vi "AES-InvCipher-text.vi"(5 "Initializer Vector":u8[](array[numeric]), 7 "Operation Mode":T1, 8 "error in (no error)":errorcluster, 10 "Cipher Key":u8[](array[numeric]), 11 "ciphertext":u8[](array[numeric])) -> (0 "error out":errorcluster, 3 "plaintext":u8[](array[numeric]))   [LabVIEW 2011, in "i3-external-encryption.lvlib"]
doc: "Decripts the <b>ciphertext</b> by using the cipher and the given <b>Operation Mode</b> using AES algorithm.\nThe cipher key and initialization vector should be a hex-string (ASCII values 0-f).\nCAUTION:\nThis VI is not secure, it does not protect the memory of the encryption, key and unencrypted data.\n\n(c) Ton Plomp, 2011\nTHIS SOFTWARE IS PROVIDED AS IS, AND ANY WARRANTY IS REJECTED"
uses:
  i3-external-encryption.lvlib
  AES-Modes.ctl
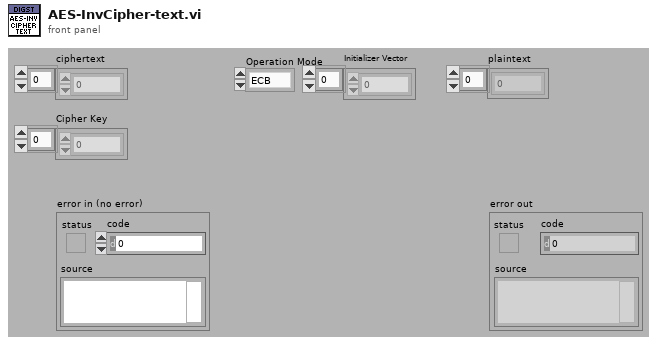
[diagram p1: front panel]
types:
  T1 = typedef "i3-external-encryption.lvlib/AES-Modes.ctl" = enum16{"ECB", "CBC", "CFB128", "OFB"}
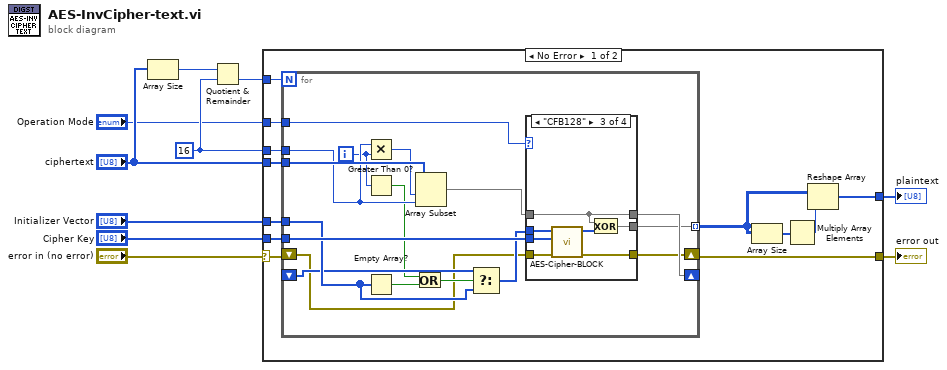
[diagram p0: block diagram]
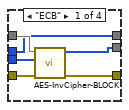
[diagram p2: hidden frame]
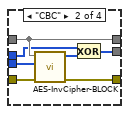
[diagram p3: hidden frame]
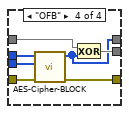
[diagram p4: hidden frame]
diagram:
  w6 = 16 ("y")
  n1 = Array Size(array="ciphertext") -> (size(s)=w8:i32)
  n2 = Quotient & Remainder(x=w8, y=w6) -> (floor(x/y)=w5:i32)  [unwired: 1 out]
  n3 = case shown="No Error" "error in (no error)" {
    selector: "error in (no error)" -> [w18 w67]
    tunnel: "ciphertext" -> [w22 _]
    tunnel: [w17 w67] -> w9
    tunnel: "Cipher Key" -> [w21 _]
    tunnel: w5 -> [w20 _]
    tunnel: w6 -> [w19 _]
    tunnel: [w11 _] -> w7
    tunnel: "Initializer Vector" -> [w15 _]
    tunnel: "Operation Mode" -> [w16 _]
    frame No Error {
      n4 = for {
        N: w20 -> [_]
        tunnel: w22 -> [w38]
        tunnel: w21 -> [w39]
        tunnel: w19 -> [w36]
        shift-right: [w33] -> w17
        shift-left: w18 -> [w25]
        tunnel: [w23] -> w12 mode=indexing
        shift-right: [w34] -> _
        shift-left: _ -> [w31]
        tunnel: w16 -> [w35]
        tunnel: w15 -> [w32]
        i -> [w29]
        n5 = Multiply(x=w36, y=w29) -> (x*y=w37:i32)
        n6 = Greater Than 0?(x=w29) -> (x > 0?=w28:bool)
        n7 = Empty Array?(array=w32) -> (empty?=w27:bool)
        n8 = Or(x=w28, y=w27) -> (x .or. y?=w26:bool)
        n9 = Array Subset(array=w38, index=w37, length=w36) -> (w24:u8[])
        n10 = Select(t=w31, s=w26, f=w32) -> (s? t:f=w30:u8[])
        n11 = case shown="\"CFB128\"" w35 {
          tunnel: w39 -> [w45 w52 w59 w66]
          tunnel: w24 -> [w44 w49 w53 w61]
          tunnel: w25 -> [w43 w51 w58 w65]
          tunnel: [w42 w46 w55 w63] -> w23
          tunnel: [w41 w50 w57 w64] -> w33
          tunnel: w30 -> [w40 w48 w54 w62]
          tunnel: [w40 w49 w53 w60] -> w34
          frame "ECB" {
            n12 = call "AES-InvCipher-BLOCK.vi"("error in (no error)"=w43, "Cipher Key"=w45, "cipher [U8]"=w44) -> ("error out"=w41:errorcluster, "plain [U8]"=w42:u8[])  [unwired: 7 in]
          }
          frame "CBC" {
            n13 = call "AES-InvCipher-BLOCK.vi"("error in (no error)"=w51, "Cipher Key"=w52, "cipher [U8]"=w49) -> ("error out"=w50:errorcluster, "plain [U8]"=w47:u8[])  [unwired: 7 in]
            n14 = Exclusive Or(1:w47, 2:w48) -> (0:w46:u8[])
          }
          frame "CFB128" {
            n15 = call "AES-Cipher-BLOCK.vi"("error in (no error)"=w58, "Cipher Key"=w59, "Plain [U8]"=w54) -> ("error out"=w57:errorcluster, "cipher [U8]"=w56:u8[])  [unwired: 7 in]
            n16 = Exclusive Or(1:w56, 2:w53) -> (0:w55:u8[])
          }
          frame "OFB" {
            n17 = call "AES-Cipher-BLOCK.vi"("error in (no error)"=w65, "Cipher Key"=w66, "Plain [U8]"=w62) -> ("error out"=w64:errorcluster, "cipher [U8]"=w60:u8[])  [unwired: 7 in]
            n18 = Exclusive Or(1:w60, 2:w61) -> (0:w63:u8[])
          }
        }
      }
      n19 = Array Size(array=w12) -> (size(s)=w14:i32[])
      n20 = Multiply Array Elements(1:w14) -> (0:w13:i32)
      n21 = Reshape Array(w12, w13) -> (w11:u8[])
    }
    frame Error {
    }
  }
  "error out" <- w9
  "plaintext" <- w7
